vi "LJM_GetHostTick32Bit.vi"() -> (1 "Tick as 2 Integers [us]":cluster{"TickUpper":u32, "TickLower":u32}, 2 "Tick Ext [us]":ext format="%#.0f", 3 "Tick Ext [ms]":ext format="%.3f")   [LabVIEW 2024]
uses:
  labjackm.dll
panel:
  # "Returns this computer's system tick count with microsecond resolution."
  # "This is an extended precision float.  The\nonly data type in LabVIEW 7.1 that will\nhold a 64-bit integer.\n\n\n\nThis is the same value split into 2\nunsigned 32-bit integers."
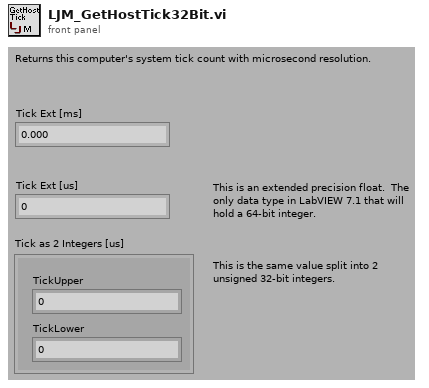
[diagram p1: front panel]
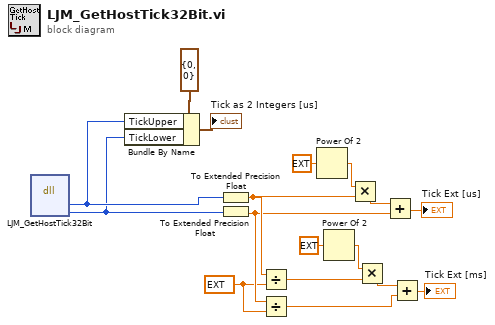
[diagram p0: block diagram]
diagram:
  w3 = ext 1000.0 ("y")
  n1 = dll-call lib="labjackm.dll" fn="LJM_GetHostTick32Bit"() -> ("TickUpper"=w11:u32, "TickLower"=w10:u32)  [unwired: 6 in, 2 out]
  n2 = Bundle By Name(cluster=cluster{"TickUpper":u32, "TickLower":u32} {"TickUpper"=0, "TickLower"=0} ("Number as 2 Integers"), "TickUpper"=w11, "TickLower"=w10) -> (→"Tick as 2 Integers [us]":cluster{"TickUpper":u32, "TickLower":u32})
  n3 = To Extended Precision Float(1:w11) -> (0:w5:ext)
  n4 = To Extended Precision Float(1:w10) -> (0:w4:ext)
  n5 = Divide(x=w5, y=w3) -> (x/y=w2:ext)
  n6 = Divide(x=w4, y=w3) -> (x/y=w1:ext)
  n7 = Power Of 2(x=ext 32.0) -> (2^x=w16:ext)
  n8 = Power Of 2(x=ext 32.0) -> (2^x=w8:ext)
  n9 = Multiply(x=w16, y=w5) -> (x*y=w15:ext)
  n10 = Multiply(x=w8, y=w2) -> (x*y=w9:ext)
  n11 = Add(x=w15, y=w4) -> (x+y=→"Tick Ext [us]":ext)
  n12 = Add(x=w9, y=w1) -> (x+y=→"Tick Ext [ms]":ext)
